vi "motor selection.vi"(0 "index 2":i32) -> (20 "[0]":bool, 21 "[1]":bool, 22 "[2]":bool, 23 "[3]":bool, 24 "[4]":bool, 25 "[5]":bool, 26 "[6]":bool, 27 "[7]":bool)   [LabVIEW 2015]
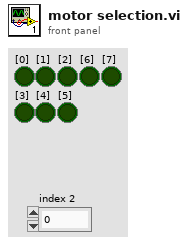
[diagram p1: front panel]
types:
  T1 = cluster{"[0]":bool, "[1]":bool, "[2]":bool, "[3]":bool, "[4]":bool, "[5]":bool, "[6]":bool, "[7]":bool, "[8]":bool}
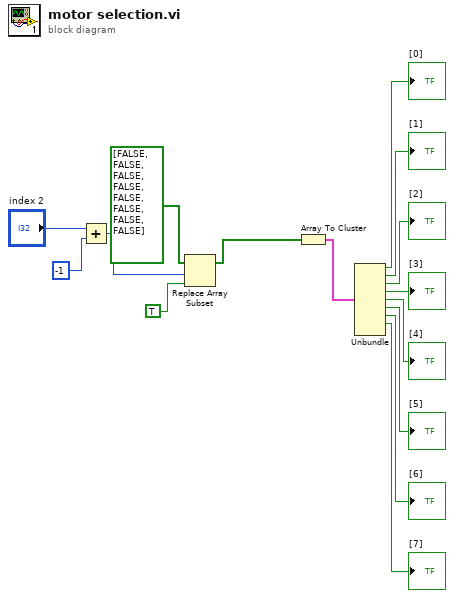
[diagram p0: block diagram]
diagram:
  n1 = Add(x="index 2", y=-1) -> (x+y=w1:i32)
  n2 = Replace Array Subset(array=bool[] [FALSE, FALSE, FALSE, FALSE, FALSE, FALSE, FALSE, FALSE], new element=TRUE, index=w1) -> (w13:bool[])
  n3 = Array To Cluster(array=w13) -> (cluster=w12:T1)
  n4 = Unbundle(w12) -> ("[0]"=→"[0]":bool, "[1]"=→"[1]":bool, "[2]"=→"[2]":bool, "[3]"=→"[3]":bool, "[4]"=→"[4]":bool, "[5]"=→"[5]":bool, "[6]"=→"[6]":bool, "[7]"=→"[7]":bool)  [unwired: 1 out]
